vi "Lab6_Spectrum_Analyzer.vi"() -> ()   [LabVIEW 2014]
uses:
  <vilib>/Analysis/4window.llb/windowTd.ctl
  <vilib>/DAQmx/create/channels.llb/DAQmx Create Channel (AI-Voltage-Basic).vi
  <vilib>/DAQmx/configure/timing.llb/DAQmx Timing (Sample Clock).vi
  <vilib>/DAQmx/read.llb/DAQmx Read (Analog Wfm 1Chan NSamp).vi
  <vilib>/measure/maspectr.llb/FFT Power Spectrum and PSD for 1 Chan.vi
  <vilib>/measure/NI_MAPro.lvlib
  <vilib>/measure/NI_MABase.lvlib
  <vilib>/Analysis/NI_AALPro.lvlib
panel:
  out "RMS dBV":dbl
  out "RMS":dbl
  out "Peak to Peak":dbl
  in  "rate":dbl=1000.0 format="%0.2f"
  out "Signal":waveform(dbl)(graph)
  in  "averaging parameters":T1={"averaging mode"=enum."No averaging", "weighting mode"=enum."Exponential", "number of averages"=10} {"number of averages" min=1}
  in  "dB On (F)":bool
  in  "window":T2=1 items=["Rectangle"=0, "Hanning"=1, "Hamming"=2, "Blackman-Harris"=3, "Exact Blackman"=4, "Blackman"=5, "Flat Top"=6, "4 Term B-Harris "=7, "7 Term B-Harris"=8, "Low Sidelobe"=9, "Blackman Nuttall"=11, "Triangle"=30, "Bartlett-Hanning"=31, "Bohman"=32, "Parzen"=33, "Welch"=34, "Kaiser"=60, "Dolph-Chebyshev"=61, "Gaussian"=62]
  in  "stop":bool
  in  "number of samples per channel":i32=-1
  out "Spectrum":cluster{"f0":dbl, "df":dbl, "magnitude":dbl[]}(graph)
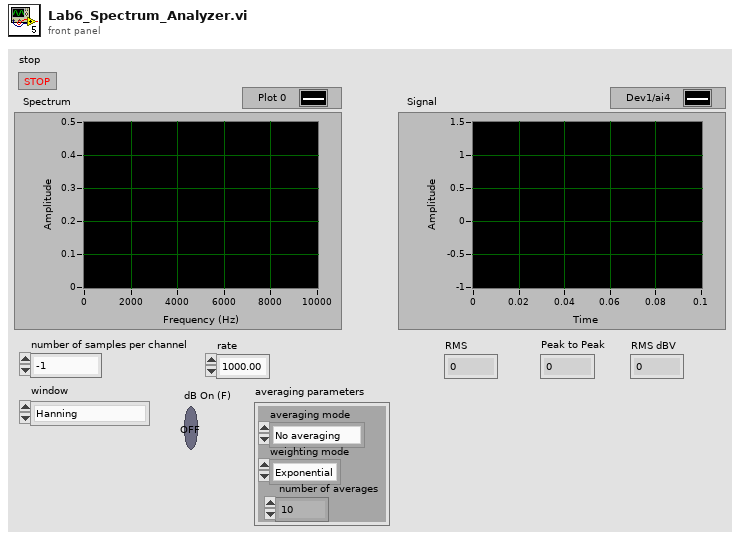
[diagram p1: front panel]
types:
  T1 = cluster{"averaging mode":enum16{"No averaging", "Vector averaging", "RMS averaging", "Peak hold"}, "weighting mode":enum16{"Linear", "Exponential"}, "number of averages":u32}
  T2 = typedef "NI_AALPro.lvlib/windowTd.ctl" = u32
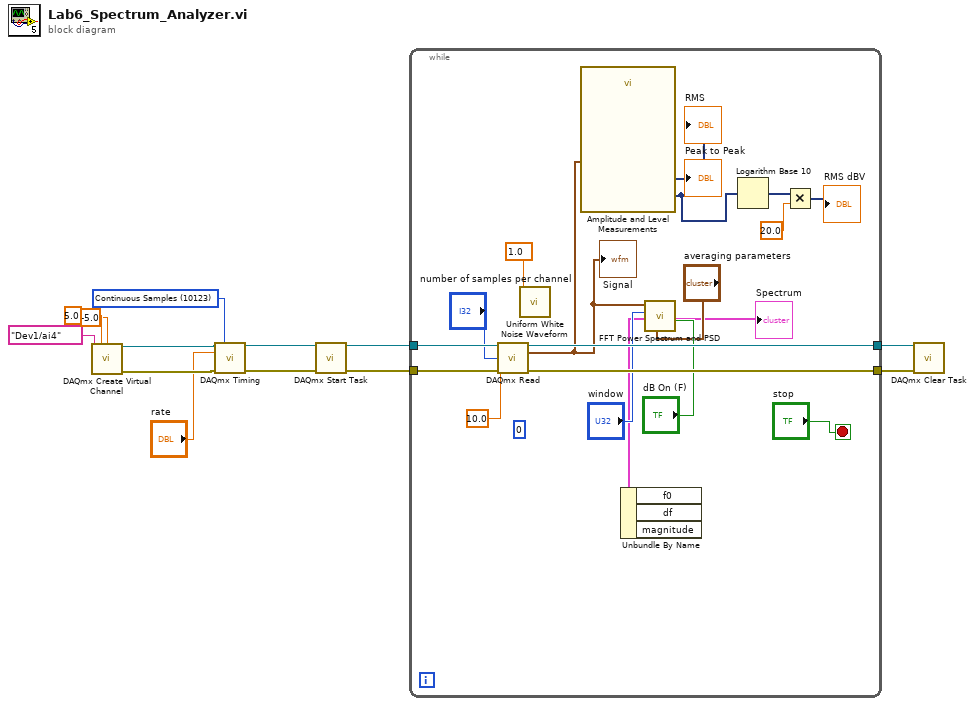
[diagram p0: block diagram]
diagram:
  w9 = 10123 items=["Finite Samples"=10178, "Continuous Samples"=10123, "Hardware Timed Single Point"=12522] ("sample mode")
  n1 = call-poly <vilib>:"DAQmx Create Virtual Channel.vi"("maximum value"=5.0, "minimum value"=-5.0, "physical channels"=tag "Dev1/ai4") -> ("task out"=w10:refnum<k21>, "error out"=w6:errorcluster)  [unwired: 11 in]
  n2 = call-poly <vilib>:"DAQmx Timing.vi"("task/channels in"=w10, "sample mode"=w9, "rate"="rate", "error in"=w6) -> ("task out"=w8:refnum<k21>, "error out"=w5:errorcluster)  [unwired: 10 in]
  n3 = call <vilib>:"DAQmx Start Task.vi"("task/channels in"=w8, "error in"=w5) -> ("task out"=w7:refnum<k21>, "error out"=w4:errorcluster)  [unwired: 12 in]
  n4 = while {
    tunnel: w7 -> [w31]
    tunnel: w4 -> [w28]
    tunnel: [w27] -> w3
    tunnel: [w26] -> w2
    stop <- "stop" stop-if-true
    (unwired) 0 ("seed")
    n5 = call-poly <vilib>:"DAQmx Read.vi"("task/channels in"=w31, "number of samples per channel"="number of samples per channel", "timeout"=10.0, "error in"=w28) -> ("task out"=w27:refnum<k21>, "data"=w15:waveform(dbl), "error out"=w26:errorcluster)  [unwired: 9 in]
    "Signal" <- w15
    n6 = call <vilib>:"Uniform White Noise Waveform.vi"("amplitude"=1.0) -> ()  [unwired: 9 in, 2 out]
    n7 = call "Amplitude and Level Measurements"("Signals"=w15) -> ("RMS"=w20:dynamicdata, "Peak to Peak"=→"Peak to Peak":dynamicdata)  [unwired: 12 in, 1 out]
    "RMS" <- w20
    n8 = call-poly <vilib>:"FFT Power Spectrum and PSD.vi"("averaging parameters"="averaging parameters", "dB On (F)"="dB On (F)", "window"="window", "time signal"=w15) -> ("Power Spectrum / PSD"=w14:cluster{"f0":dbl, "df":dbl, "magnitude":dbl[]})  [unwired: 4 in, 3 out]
    "Spectrum" <- w14
    n9 = Unbundle By Name(w14) -> ()  [unwired: 3 out]
    n10 = Logarithm Base 10(1:w20) -> (0:w19:dynamicdata)
    n11 = Multiply(x=w19, y=20.0) -> (x*y=→"RMS dBV":dynamicdata)
  }
  n12 = call <vilib>:"DAQmx Clear Task.vi"("task in"=w3, "error in"=w2) -> ()  [unwired: 13 in, 1 out]
